vi "Global Varibal Control.vi"() -> ()   [LabVIEW 2020]
uses:
  Type Definitions.llb/3 way Status.ctl
panel:
  in  "Temp (K)":dbl format="%.2f"
  in  "Previous Experiment Status":T2 {"Exposure" items=["N.A.", "OK", "Busy", "Done"]; "Spectrometer" items=["N.A.", "OK", "Busy", "Done"]; "Temperature" items=["N.A.", "OK", "Busy", "Done"]; "Field" items=["N.A.", "OK", "Busy", "Done"]}
  in  "Current Experiment Status":T2 {"Exposure" items=["N.A.", "OK", "Busy", "Done"]; "Spectrometer" items=["N.A.", "OK", "Busy", "Done"]; "Temperature" items=["N.A.", "OK", "Busy", "Done"]; "Field" items=["N.A.", "OK", "Busy", "Done"]}
  in  "SweepRate (T/min)":dbl=10.0 format="%.2f"
  in  "Desired Field (T)":dbl format="%.2f"
  in  "Current nm":dbl=6000.0 min=0.0 max=26000.0 format="%.2f"
  in  "Current WL":dbl=6000.0 min=0.0 max=26000.0 format="%.2f"
  in  "Current Counter Position":dbl=6000.0 min=0.0 max=26000.0 format="%.2f"
  in  "CurrentStepperPosition":i32 min=-8388607 max=8388607
  in  "Original Counter Position":dbl=6000.0 min=0.0 max=26000.0 format="%.2f"
  in  "Wavelength Unit":u8(ring)=1 items=["Point #", "nanometer (nm)", "electron volt (eV)", "Milli eV (meV)", "Wavenumber (cm-1)"]
  in  "Grating Density":u8(ring)=2 items=["150 g/mm", "300 g/mm", "600 g/mm", "1200 g/mm", "1800 g/mm"]
  in  "# of Pinned Columns":u8=5 max=10
  in  "Buffer Size":u8=100
  in  "Master Initialization?":bool=TRUE
  in  "Global Cancel":bool
  in  "Field OK":bool
  in  "PS SlewRate":dbl=200.0 format="%.2f"
  in  "PS Setpoint":dbl format="%.2f"
  in  "PS Current":dbl format="%.2f"
  in  "PowerSupply OK?":bool
  in  "PowerSupply ON?":bool
  in  "CCD OK?":bool
  in  "McP OK?":bool
  in  "McP Steps/Angstrom":i32=250 min=250 max=250
  in  "McP Port#":i32=1 min=0 max=5
  in  "McP Scan Velocity":i32
  in  "CCD Setup String":string
  # "McPherson Controls"
  # "Field Controls"
  # "CCD Controls"
  # "General Controls"
  # "Temperature"
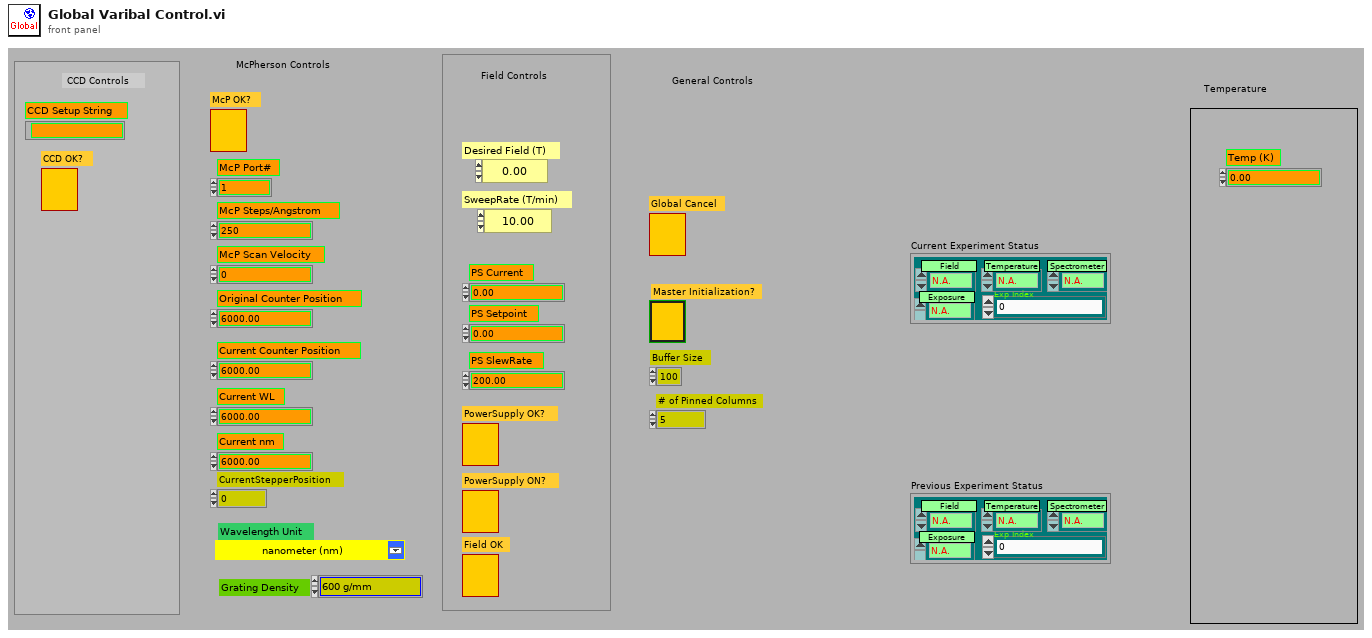
[diagram p1: front panel]
types:
  T1 = typedef "3 way Status.ctl" = u8
  T2 = cluster{"Exp Index":u32, "Field":T1, "Temperature":T1, "Spectrometer":T1, "Exposure":T1}
diagram:
